vi "sv_Init Relative Response.vi"(0 "power spectrum":cluster{"f0":dbl, "df":dbl, "Spectrum":dbl[]} {"Spectrum" format="%.2f"; "df" format="%.2f"; "f0" format="%.2f"}, 7 "weighting filter":T5 items=["Linear", "A-weighting", "B-weighting", "C-weighting", "ITU-R 468-4", "Dolby", "CCITT", "C-message", "Wb", "Wc", "Wd", "We", "Wf", "Wh", "Wj", "Wk", "Wm", "AES17 20 kHz lowpass", "AES17 40 kHz lowpass", "AES17 20 kHz highpass", "AES17 40 kHz highpass"], 9 "spectrum info":T1={"channel name"="", "description"="", "x-axis units"=0, "spectral info"={"spectrum type"=enum."Power [Magnitude^2]", "linear/dB"=enum."linear", "window"=0, "window size"=0, "FFT size"=0}, "engineering units"=0, "custom label"="", "dB reference [EU]"=0.0, "peak units"=enum."rms", "weighting filter"=0, "spectral density?"=FALSE, "unit label"="", "spectrum skewed?"=FALSE, "complimentary spectrum units"=enum."none"} {"x-axis units" items=["Time (s)"=0, "Frequency-CB (Hz)"=1, "Frequency-CPB (Hz)"=1248, "Frequency-Arbitrary (Hz)"=2357, "Quefrency (s)"=2, "Revolutions (rev)"=3, "Order"=4, "Speed (RPM)"=11, "Speed (rad/s)"=21, "Index"=65535]; "weighting filter" items=["Linear", "A-weighting", "B-weighting", "C-weighting", "ITU-R 468-4", "Dolby", "CCITT", "C-message", "Wb", "Wc", "Wd", "We", "Wf", "Wh", "Wj", "Wk", "Wm", "AES17 20 kHz lowpass", "AES17 40 kHz lowpass", "AES17 20 kHz highpass", "AES17 40 kHz highpass"]; "dB reference [EU]" format="%.2f"; "engineering units" items=["custom..."=0, "V"=1, "A"=21, "C"=30, "pC"=31, "s"=32, "-"=29, "Pa"=2, "N"=20, "g"=3, "m/s^2"=4, "m/s"=5, "m"=6, "mm/s"=12, "mm"=13, "micron/s"=14, "micron"=15, "in/s^2"=7, "in/s"=8, "in"=9, "mil/s"=10, "mil"=11, "rad/s^2"=16, "rad/s"=17, "rad"=18, "deg/s^2"=26, "deg/s"=27, "deg"=28, "RPM"=22, "cycle/s^2"=23, "Hz"=24, "cycle"=25, "strain"=19]; "spectral info"."window" items=["None "=0, "Hanning"=1, "Hamming"=2, "Blackman-Harris"=3, "Exact Blackman"=4, "Blackman"=5, "Flat Top"=6, "4 Term B-Harris "=7, "7 Term B-Harris"=8, "Low Sidelobe"=9, "Force - Exponential"=10, "Gaussian"=62]}, 11 "error in (no error)":errorcluster, 12 "reset":bool) -> (4 "dup power spectrum":cluster{"f0":dbl, "df":dbl, "Spectrum":dbl[]} {"Spectrum" format="%.2f"; "df" format="%.2f"; "f0" format="%.2f"}, 8 "relative response":dbl[](array[numeric]) format="%.2f", 10 "dup spectrum info in":T1={"channel name"="", "description"="", "x-axis units"=0, "spectral info"={"spectrum type"=enum."Power [Magnitude^2]", "linear/dB"=enum."linear", "window"=0, "window size"=0, "FFT size"=0}, "engineering units"=0, "custom label"="", "dB reference [EU]"=0.0, "peak units"=enum."rms", "weighting filter"=0, "spectral density?"=FALSE, "unit label"="", "spectrum skewed?"=FALSE, "complimentary spectrum units"=enum."none"} {"x-axis units" items=["Time (s)"=0, "Frequency-CB (Hz)"=1, "Frequency-CPB (Hz)"=1248, "Frequency-Arbitrary (Hz)"=2357, "Quefrency (s)"=2, "Revolutions (rev)"=3, "Order"=4, "Speed (RPM)"=11, "Speed (rad/s)"=21, "Index"=65535]; "weighting filter" items=["Linear", "A-weighting", "B-weighting", "C-weighting", "ITU-R 468-4", "Dolby", "CCITT", "C-message", "Wb", "Wc", "Wd", "We", "Wf", "Wh", "Wj", "Wk", "Wm", "AES17 20 kHz lowpass", "AES17 40 kHz lowpass", "AES17 20 kHz highpass", "AES17 40 kHz highpass"]; "dB reference [EU]" format="%.2f"; "engineering units" items=["custom..."=0, "V"=1, "A"=21, "C"=30, "pC"=31, "s"=32, "-"=29, "Pa"=2, "N"=20, "g"=3, "m/s^2"=4, "m/s"=5, "m"=6, "mm/s"=12, "mm"=13, "micron/s"=14, "micron"=15, "in/s^2"=7, "in/s"=8, "in"=9, "mil/s"=10, "mil"=11, "rad/s^2"=16, "rad/s"=17, "rad"=18, "deg/s^2"=26, "deg/s"=27, "deg"=28, "RPM"=22, "cycle/s^2"=23, "Hz"=24, "cycle"=25, "strain"=19]; "spectral info"."window" items=["None "=0, "Hanning"=1, "Hamming"=2, "Blackman-Harris"=3, "Exact Blackman"=4, "Blackman"=5, "Flat Top"=6, "4 Term B-Harris "=7, "7 Term B-Harris"=8, "Low Sidelobe"=9, "Force - Exponential"=10, "Gaussian"=62]}, 15 "error out":errorcluster)   [LabVIEW 2017]
uses:
  <vilib>/addons/_NISVFA/_Shared subVIs/Controls/svc_Weighting Filter Text Ring.ctl
  <vilib>/addons/_NISVFA/_Shared subVIs/Controls/svc_Spectrum Info.ctl
  <vilib>/addons/_NISVFA/_Shared subVIs/Controls/svc_X-Axis Units.ctl
  <vilib>/addons/_NISVFA/_Shared subVIs/Controls/svc_Spectrum Type.ctl
  <vilib>/addons/_NISVFA/_Shared subVIs/Controls/svc_Engineering Units Text Ring.ctl
  <vilib>/addons/_NISVFA/_Shared subVIs/Controls/svc_Complimentary Spectrum Units.ctl
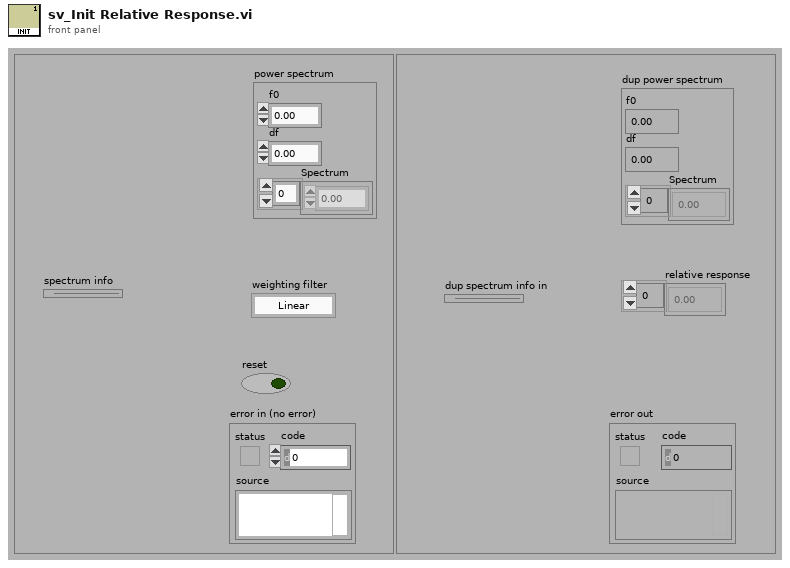
[diagram p1: front panel]
types:
  T1 = typedef "svc_Spectrum Info.ctl" = cluster{"channel name":string, "description":string, "x-axis units":T2, "spectral info":cluster{"spectrum type":T3, "linear/dB":enum16{"linear", "dB"}, "window":u16, "window size":i32, "FFT size":i32}, "engineering units":T4, "custom label":string, "dB reference [EU]":dbl, "peak units":enum16{"rms", "peak", "peak-peak"}, "weighting filter":T5, "spectral density?":bool, "unit label":string, "spectrum skewed?":bool, "complimentary spectrum units":T6}
  T2 = typedef "svc_X-Axis Units.ctl" = u16
  T3 = typedef "svc_Spectrum Type.ctl" = enum16{"FFT Spectrum [complex]", "Amplitude [Magnitude]", "Power [Magnitude^2]", "Cross Spectrum [complex]", "Frequency Response [Complex]"}
  T4 = typedef "svc_Engineering Units Text Ring.ctl" = u16
  T5 = typedef "svc_Weighting Filter Text Ring.ctl" = u16
  T6 = typedef "svc_Complimentary Spectrum Units.ctl" = enum16{"none", "radians", "degrees", "cycles", "imaginary"}
  T7 = enum16{"FFT Spectrum [complex]", "Amplitude [Magnitude]", "Power [Magnitude^2]", "Cross Spectrum [complex]", "Frequency Response [Complex]"}
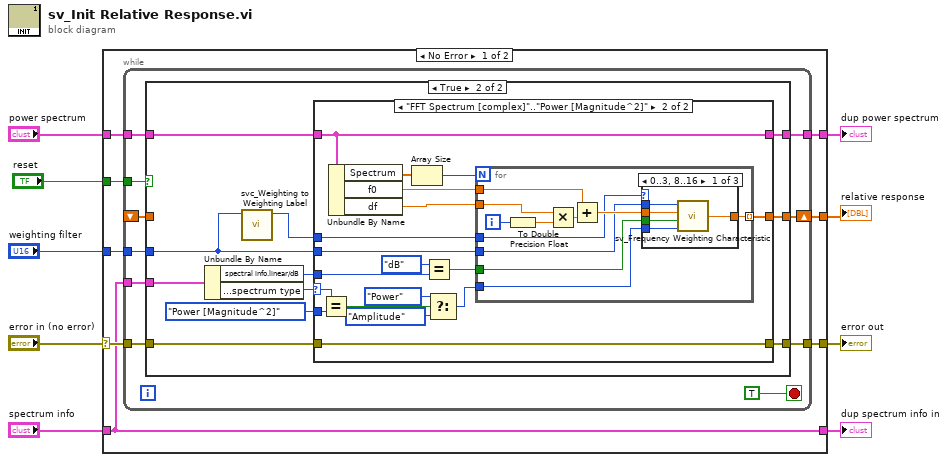
[diagram p0: block diagram]
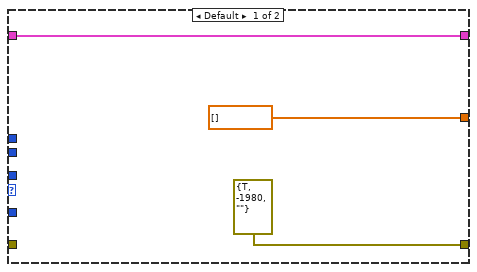
[diagram p3: hidden frame]
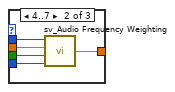
[diagram p4: hidden frame]
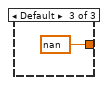
[diagram p5: hidden frame]
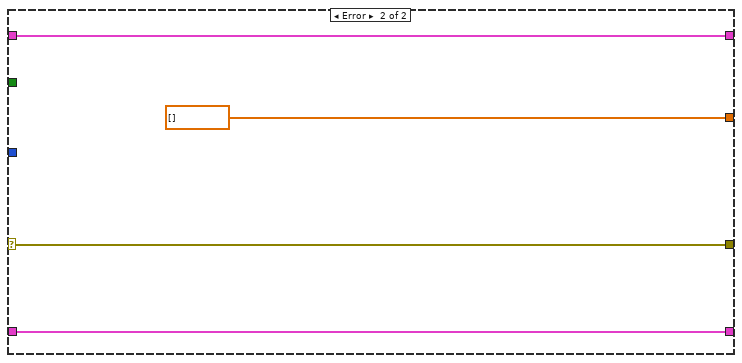
[diagram p6: hidden frame]
diagram:
  n1 = case shown="No Error" "error in (no error)" {
    selector: "error in (no error)" -> [w16 w86]
    tunnel: [w17 w86] -> w8
    tunnel: "power spectrum" -> [w15 w88]
    tunnel: [w14 w88] -> w6
    tunnel: "weighting filter" -> [w13 _]
    tunnel: "spectrum info" -> [w11 w87]
    tunnel: [w12 dbl[] []] -> w3
    tunnel: [w11 w87] -> w2
    tunnel: "reset" -> [w10 _]
    frame No Error {
      n2 = while {
        tunnel: [w27] -> w17
        tunnel: w16 -> [w26]
        tunnel: w15 -> [w25]
        tunnel: [w24] -> w14
        tunnel: w11 -> [w23]
        tunnel: w13 -> [w22]
        shift-right: [w21] -> w12
        shift-left: _ -> [w19]
        tunnel: w10 -> [w20]
        stop <- TRUE stop-if-true
        n3 = case shown="True" w20 {
          tunnel: [w28 w40] -> w27
          tunnel: w26 -> [w28 w38]
          tunnel: w25 -> [w30 w37]
          tunnel: [w30 w36] -> w24
          tunnel: w23 -> [_ w35]
          tunnel: w22 -> [_ w33]
          tunnel: [w29 w31] -> w21
          tunnel: w19 -> [w29 _]
          frame False {
          }
          frame True {
            n4 = Unbundle By Name(w35) -> ("spectral info.linear/dB"=w34:enum16{"linear", "dB"}, "spectral info.spectrum type"=w41:T3)
            n5 = call <vilib>:"svc_Weighting to Weighting Label.vi"("weighting filter"=w33) -> ("weighting enum"=w32:T5)  [unwired: 9 in, 1 out]
            n6 = case shown="\"FFT Spectrum [complex]\"..\"Power [Magnitude^2]\"" w41 {
              selector: w41 -> [_ w53]
              tunnel: [dbl[] [] w55] -> w31
              tunnel: w37 -> [w44 w56]
              tunnel: w33 -> [_ w58]
              tunnel: [errorcluster {"status"=TRUE, "code"=-1980, "source"=""} ("error IO") w57] -> w40
              tunnel: T7."Power [Magnitude^2]" ("y") -> [_ w54]
              tunnel: w38 -> [_ w57]
              tunnel: [w44 w56] -> w36
              tunnel: w34 -> [_ w48]
              tunnel: w32 -> [_ w45]
              frame Default {
              }
              frame "FFT Spectrum [complex]".."Power [Magnitude^2]" {
                n7 = Equal?(x=w53, y=w54) -> (x = y?=w52:bool)
                n8 = Unbundle By Name(w56) -> ("Spectrum"=w61:dbl[], "f0"=w60:dbl, "df"=w59:dbl)
                n9 = Array Size(array=w61) -> (size(s)=w62:i32)
                n10 = Equal?(x=enum16{"linear", "dB"}."dB" ("y"), y=w48) -> (x = y?=w46:bool)
                n11 = Select(t=enum16{"Power", "Amplitude"}."Power" ("spectrum type"), s=w52, f=enum16{"Power", "Amplitude"}."Amplitude" ("spectrum type")) -> (s? t:f=w51:enum16{"Power", "Amplitude"})
                n12 = for {
                  N: w62 -> [_]
                  tunnel: [w72] -> w55 mode=indexing
                  tunnel: w60 -> [w69]
                  tunnel: w59 -> [w67]
                  tunnel: w58 -> [w66]
                  tunnel: w51 -> [w65]
                  tunnel: w46 -> [w64]
                  tunnel: w45 -> [w63]
                  i -> [w73]
                  n13 = To Double Precision Float(number=w73) -> (double precision float=w71:dbl)
                  n14 = Multiply(x=w67, y=w71) -> (x*y=w68:dbl)
                  n15 = Add(x=w69, y=w68) -> (x+y=w70:dbl)
                  n16 = case shown="0..3, 8..16" w63 {
                    tunnel: [w78 w79 nan ("relative response level")] -> w72
                    tunnel: w70 -> [w77 w82 _]
                    tunnel: w66 -> [w76 w83 _]
                    tunnel: w65 -> [w75 w80 _]
                    tunnel: w64 -> [w74 w81 _]
                    frame 0..3, 8..16 {
                      n17 = call <vilib>:"sv_Frequency Weighting Characteristic.vi"("spectrum type"=w75, "dB On (T)"=w74, "frequency [Hz]"=w77, "weighting filter"=w76) -> ("relative response level"=w78:dbl)
                    }
                    frame 4..7 {
                      n18 = call <vilib>:"sv_Audio Frequency Weighting.vi"("spectrum type"=w80, "dB On (T)"=w81, "frequency [Hz]"=w82, "weighting filter"=w83) -> ("relative response level"=w79:dbl)
                    }
                    frame Default {
                    }
                  }
                }
              }
            }
          }
        }
      }
    }
    frame Error {
    }
  }
  "error out" <- w8
  "dup power spectrum" <- w6
  "relative response" <- w3
  "dup spectrum info in" <- w2
